vi "Complex Test.vi"() -> ()   [LabVIEW 2020, in "infolib.lvlib"]
doc: "Make a complex test of the library using premade tests/test.info."
uses:
  infolib.lvlib
  GetString.vi
  String.vi
  Get 2D String.vi
  2D String.vi
  GetTime Stamp.vi
  Time Stamp.vi
  Get 2D Time Stamp.vi
  2D Time Stamp.vi
  GetEXT.vi
  EXT.vi
  GetCXT.vi
  CXT.vi
  Get 2D EXT.vi
  2D EXT.vi
  Get 2D CXT.vi
  2D CXT.vi
  <vilib>/Utility/error.llb/Error Cluster From Error Code.vi
  <vilib>/ErrorRing/Error Ring.xnode
panel:
  in  "Test definitions and correct values":T1(array[cluster])=[{"k"="Test key, no value", "v"=[[""]], "t"="string", "s"=[]}, {"k"="Test key", "v"=[["A"]], "t"="string", "s"=[]}, {"k"="Test key, similar", "v"=[["B"]], "t"="string", "s"=[]}, {"k"="Test key, no spaces", "v"=[["C"]], "t"="string", "s"=[]}, {"k"="Test key, both spaces", "v"=[["D"]], "t"="string", "s"=[]}, {"k"="Test key, space left", "v"=[["E"]], "t"="string", "s"=[]}, {"k"="Test key, space right", "v"=[["F"]], "t"="string", "s"=[]}, {"k"="Test integer, 16 digits", "v"=[["1234567890123456"]], "t"="number", "s"=[]}, {"k"="Test floating point, 16 digits after decimal dot", "v"=[["0.1234567890123456"]], "t"="number", "s"=[]}, {"k"="Test floating point, 15 digits before decimal dot", "v"=[["123456789012345.6"]], "t"="number", "s"=[]}, {"k"="Test complex number", "v"=[["2.34+5.67i"]], "t"="compl. number", "s"=[]}, {"k"="Test imaginary number", "v"=[["8.90i"]], "t"="compl. number", "s"=[]}, {"k"="Test string, simple", "v"=[["test string"]], "t"="string", "s"=[]}, {"k"="Test string, nonletter characters", "v"=[["!@#$%^&*()-=[]{};'\"\\'\\\"\\:|,./<>?"]], "t"="string", "s"=[]}, {"k"="Test string, nonletter characters in key !@#$%^&*()-=[]{};'\"\\'\\\"\\:|,./<>?", "v"=[["in key"]], "t"="string", "s"=[]}, {"k"="Test string, UTF8 characters", "v"=[["\\u0159\\u0153\\u0414\\u03bc\\u03a9\\u211c\\u2111"]], "t"="string", "s"=[]}, {"k"="Test string, UTF8 characters in key \\u0159\\u0153\\u0414\\u03bc\\u03a9\\u211c\\u2111", "v"=[["in key"]], "t"="string", "s"=[]}, {"k"="Test time, no time zone", "v"=[["1014376332.123456"]], "t"="time", "s"=[]}, {"k"="Test time, with time zone, UTC", "v"=[["1014379932.123456"]], "t"="time", "s"=[]}, {"k"="Test time, with time zone, +10 minutes", "v"=[["1014379932.123456"]], "t"="time", "s"=[]}, {"k"="Test time, with time zone, +1 hour", "v"=[["1014379932.123456"]], "t"="time", "s"=[]}, {"k"="Test time, with time zone, -1 hour", "v"=[["1014379932.123456"]], "t"="time", "s"=[]}, {"k"="Test time, with time zone, +1:10", "v"=[["1014379932.123456"]], "t"="time", "s"=[]}, {"k"="Test time, with time zone, -1:10", "v"=[["1014379932.123456"]], "t"="time", "s"=[]}, {"k"="Test matrix, empty", "v"=[[""]], "t"="matrix number", "s"=[]}, {"k"="Test matrix, single value", "v"=[["1"]], "t"="matrix number", "s"=[]}, {"k"="Test matrix, single value, nonletter characters in key !@#$%^&*()-=[]{};'\"\\'\\\"\\:|,./<>?", "v"=[["2"]], "t"="matrix number", "s"=[]}, {"k"="Test matrix, single value, UTF8 characters in key  \\u0159\\u0153\\u0414\\u03bc\\u03a9\\u211c\\u2111", "v"=[["3"]], "t"="matrix number", "s"=[]}, {"k"="Test matrix, row numbers", "v"=[["4", "5", "6"]], "t"="matrix number", "s"=[]}, {"k"="Test matrix, column numbers", "v"=[["7"], ["8"], ["9"]], "t"="matrix number", "s"=[]}, {"k"="Test matrix", "v"=[["1.1", "2.1", "3.1"], ["4e4", "-5e5", "6e-6"], ["7.7e7", "8.123456789e1", "NaN"]], "t"="matrix number", "s"=[]}, {"k"="Test matrix complex", "v"=[["1.234", "2.345i", "3.456+4.567i"]], "t"="matrix compl. number", "s"=[]}, {"k"="Test matrix, mixed numbers and text for reading as numbers", "v"=[["1", "NaN", "2", "NaN"], ["3", "NaN", "4", "NaN"]], "t"="matrix number", "s"=[]}, {"k"="Test matrix, mixed numbers and text for reading as strings", "v"=[["11", "One", "12", "Two"], ["13", "Three", "14", "Four"]], "t"="matrix string", "s"=[]}, {"k"="Test matrix, mixed numbers and text with special characters read as numbers", "v"=[["1", "NaN", "2", "NaN"], ["3", "NaN", "4", "NaN"]], "t"="matrix number", "s"=[]}, {"k"="Test matrix, mixed numbers and text with special characters read as strings", "v"=[["11", "One;One", "12", "Two\"Two"], ["13", "Three;Three", "14", "Four\n                Four"]], "t"="matrix string", "s"=[]}, {"k"="Test matrix, time values", "v"=[["1014379932.123456", "1014383532.123456"], ["1014387132.123456", "1014390732.123456"]], "t"="matrix time", "s"=[]}, {"k"="Key for section test", "v"=[["1"]], "t"="number", "s"=[""]}, {"k"="Key for section test", "v"=[["2"]], "t"="number", "s"=["Test section"]}, {"k"="Key for section test", "v"=[["3"]], "t"="number", "s"=["Test section", "Test subsection"]}, {"k"="Key for section test", "v"=[["4"]], "t"="number", "s"=["Test section", "Test subsection", "Test subsubsection"]}, {"k"="Key for section test", "v"=[["5"]], "t"="number", "s"=["Test section", "Test subsection", "Test subsubsection", "Test subsubsubsection"]}, {"k"="Key for section test", "v"=[["6"]], "t"="number", "s"=["Test section 2"]}, {"k"="Key for section test", "v"=[["7"]], "t"="number", "s"=["Test section 2", "Test section 2"]}, {"k"="Key for section test", "v"=[["8"]], "t"="number", "s"=["Test section 2", "Test section 2", "Test section 2"]}, {"k"="Key for section test", "v"=[["9"]], "t"="number", "s"=["Test section 2", "Test section 2", "Test section 2", "Test section 2"]}, {"k"="Key for section test", "v"=[["10"]], "t"="number", "s"=["Test section, nonletter characters in key !@#$%^&*()-=[]{};'\"\\'\\\"\\:|,./<>?"]}, {"k"="Key for section test", "v"=[["11"]], "t"="number", "s"=["Test section, UTF8 characters in key \\u0159\\u0153\\u0414\\u03bc\\u03a9\\u211c\\u2111"]}, {"k"="Key for section test", "v"=[["!@#$%^&*()-=[]{};'\"\\'\\\"\\:|,./<>?"]], "t"="section", "s"=["Test section, special characters inside"]}]
  in  "Do also tmp.info?":bool=TRUE
  in  "start:":i32
  in  "end:":i32=100
  out "tmp.info: all correct?":bool
  out "tmp.info: all keys found?":bool
  out "Results of testing":T2(array[cluster])
  out "test.info: all keys found?":bool
  out "test.info: all correct?":bool
  # "k: key, v: value of correct value, t: test type, s: section(s)"
  # "For details see \"tests/info_test.m\" and \"tests/test.info\"."
  # "Do not change values in the array without changing test.info and other testing scripts (infolib_test.m)!"
  # "First run from test.info"
  # "test index, test key, key found?, test correct?"
  # "Second run from generated tmp.info"
  # "For debugging: do tests only from index"
  # "to index"
  # "(inclusive), do tmp.info"
  # "<- To make full test, set values to 0 and 100 and check tmp.info."
  # "List of bad tests, with very small impact:\n15, 16, 27, 47, 48: LV cannot handle UTF8 characters\n43: fails if tests 47 and 48 are present in tmp.info, otherwise is ok.\n30: rounding error on 17th significant place\n34,:LV cannot handle proper csv: cell \"X;X\" is considered as two cells because LV do not know apostroph enclosing\n36: rounding error on 7th decimal place of time stamp"
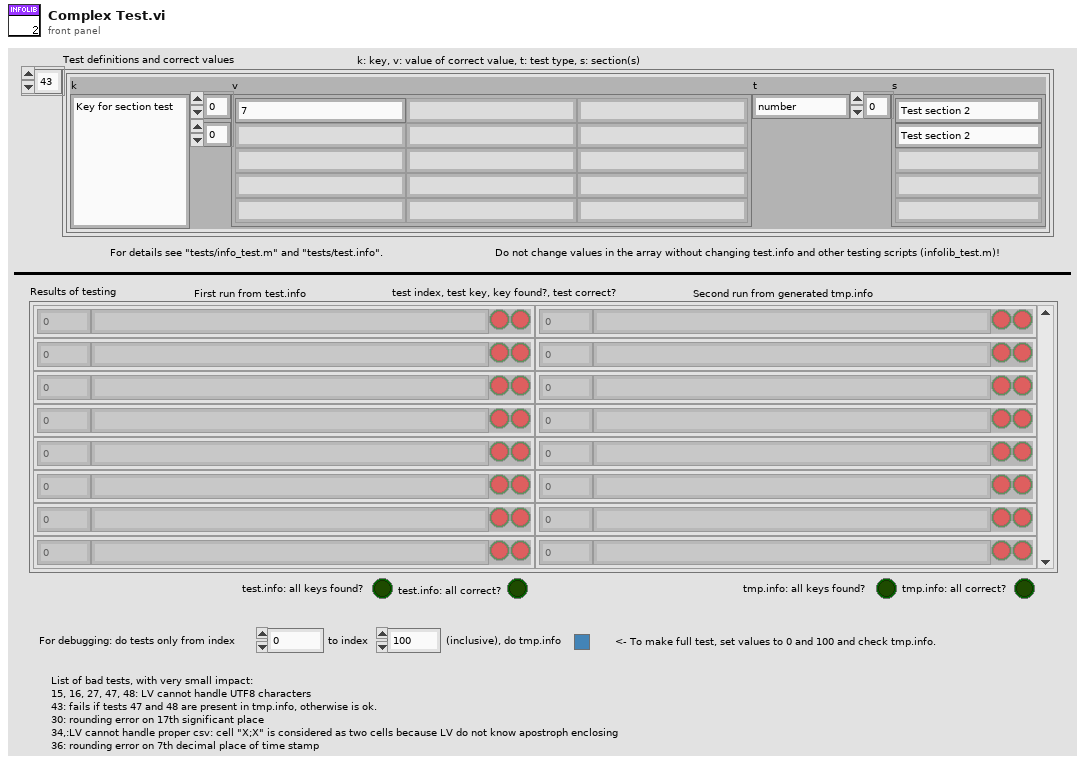
[diagram p1: front panel]
types:
  T1 = cluster{"k":string, "v":string[][], "t":string, "s":string[]}[]
  T2 = cluster{"index":i32, "key":string, "key found?":bool, "correct?":bool}[][]
  T3 = cluster{"index":i32, "key":string, "key found?":bool, "correct?":bool}
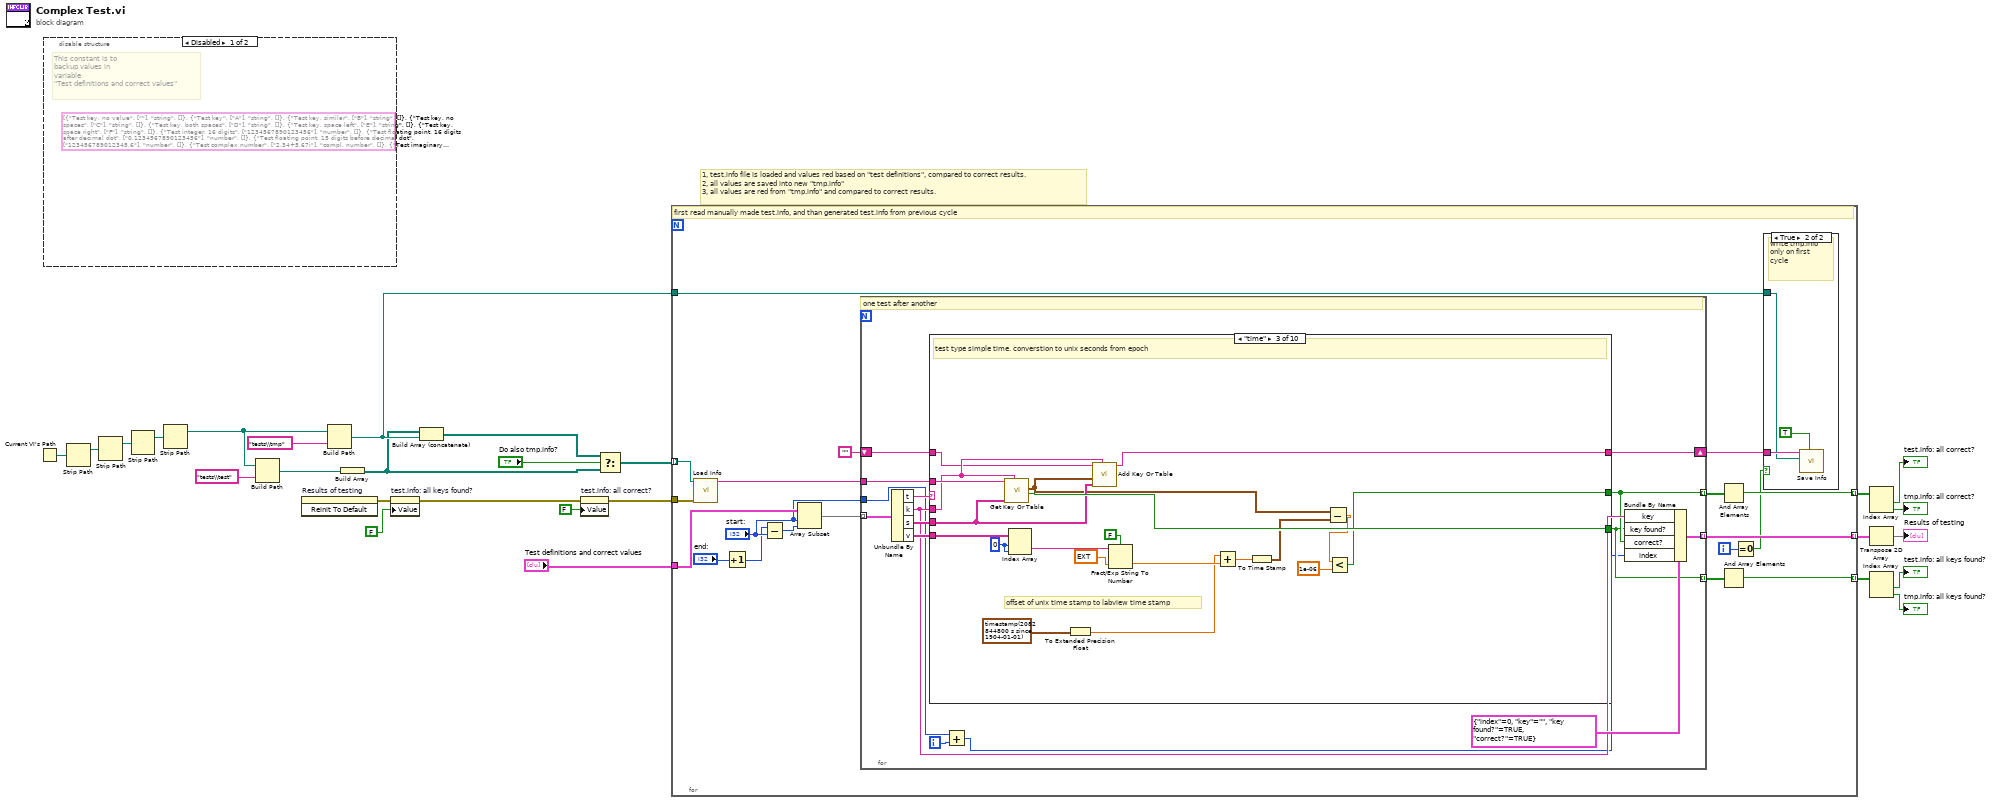
[diagram p0: block diagram]
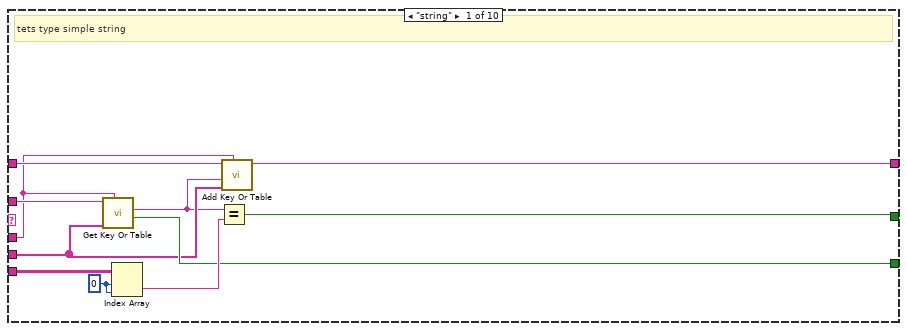
[diagram p3: hidden frame]
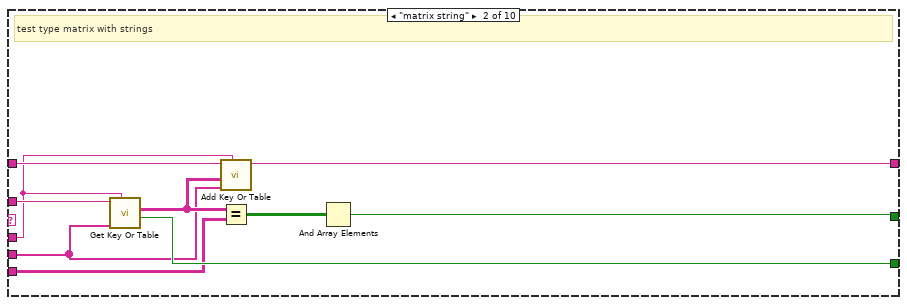
[diagram p4: hidden frame]
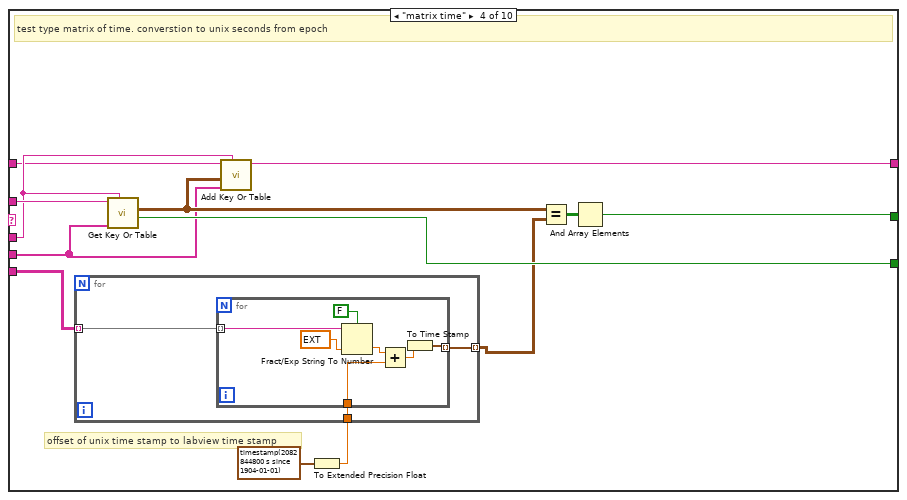
[diagram p5: hidden frame]
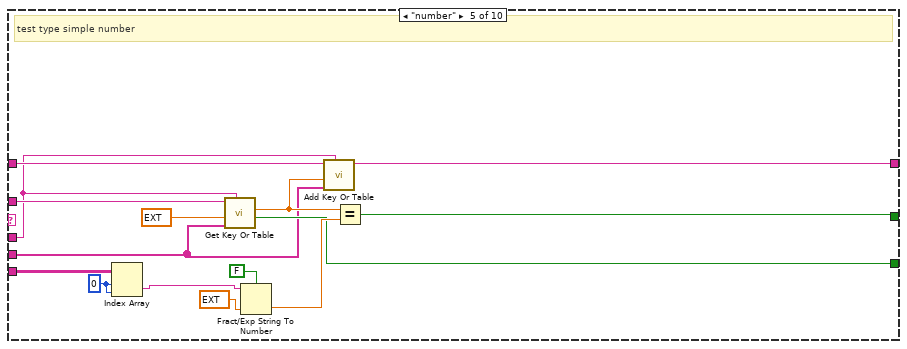
[diagram p6: hidden frame]
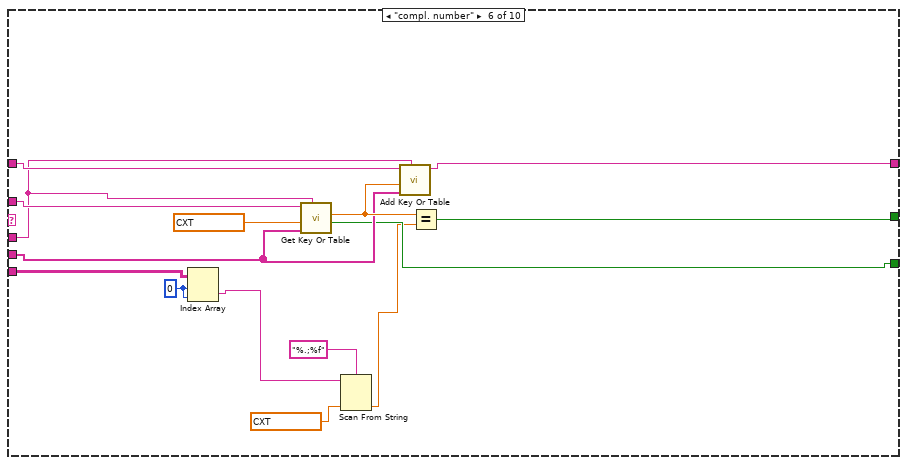
[diagram p7: hidden frame]
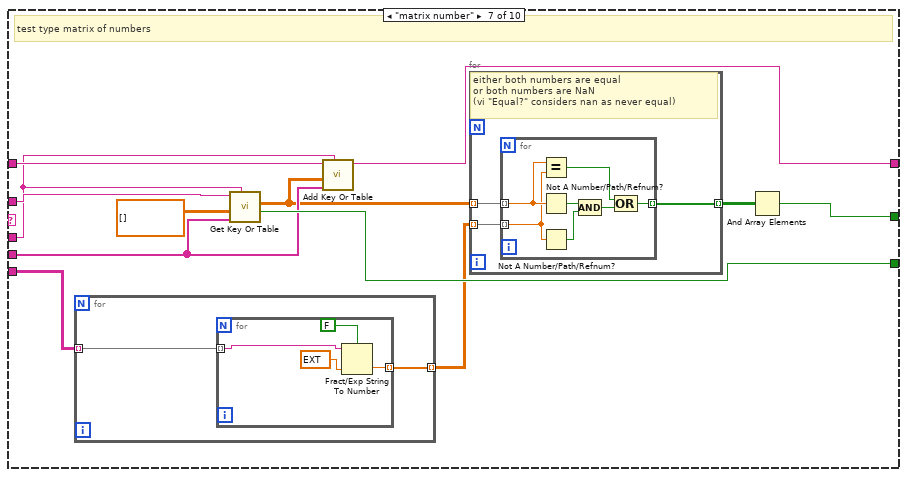
[diagram p8: hidden frame]
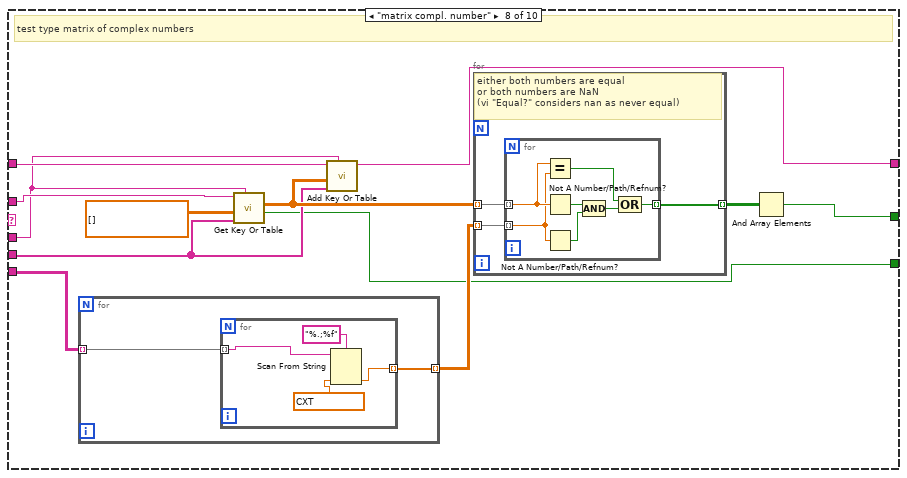
[diagram p9: hidden frame]
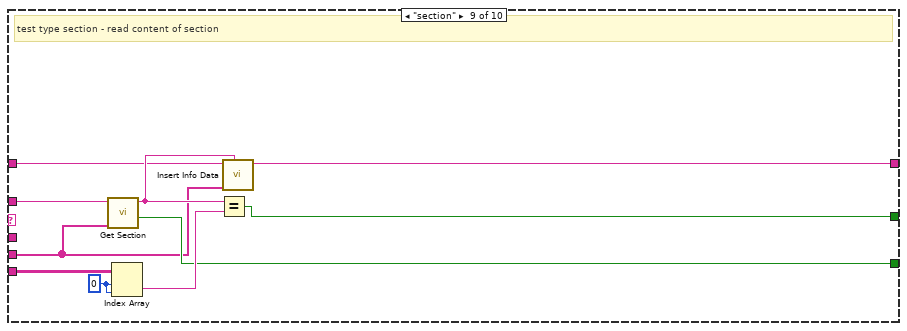
[diagram p10: hidden frame]
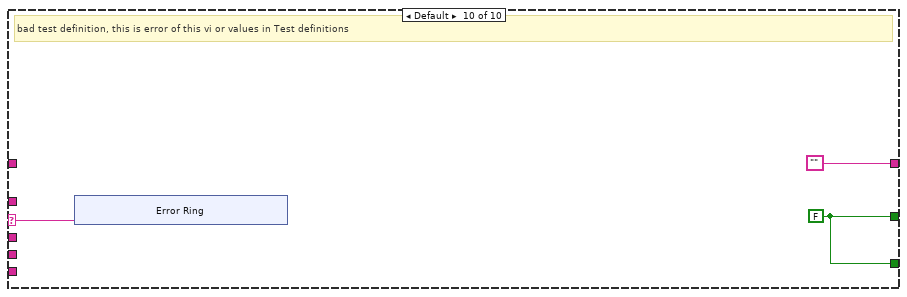
[diagram p11: hidden frame]
diagram:
  # "1, test.info file is loaded and values red based on \"test definitions\", compared to correct results.\n2, all values are saved into new \"tmp.info\"\n3, all values are red from \"tmp.info\" and compared to correct results."
  n1 = Current VI's Path() -> (path=w15:path)
  n2 = disable-structure shown="Disabled" {
    frame Disabled {
      (unwired) T1 [{"k"="Test key, no value", "v"=[[""]], "t"="string", "s"=[]}, {"k"="Test key", "v"=[["A"]], "t"="string", "s"=[]}, {"k"="Test key, similar", "v"=[["B"]], "t"="string", "s"=[]}, {"k"="Test key, no spaces", "v"=[["C"]], "t"="string", "s"=[]}, {"k"="Test key, both spaces", "v"=[["D"]], "t"="string", "s"=[]}, {"k"="Test key, space left", "v"=[["E"]], "t"="string", "s"=[]}, {"k"="Test key, space right", "v"=[["F"]], "t"="string", "s"=[]}, {"k"="Test integer, 16 digits", "v"=[["1234567890123456"]], "t"="number", "s"=[]}, {"k"="Test floating point, 16 digits after decimal dot", "v"=[["0.1234567890123456"]], "t"="number", "s"=[]}, {"k"="Test floating point, 15 digits before decimal dot", "v"=[["123456789012345.6"]], "t"="number", "s"=[]}, {"k"="Test complex number", "v"=[["2.34+5.67i"]], "t"="compl. number", "s"=[]}, {"k"="Test imaginary number", "v"=[["8.90i"]], "t"="compl. number", "s"=[]}, {"k"="Test string, simple", "v"=[["test string"]], "t"="string", "s"=[]}, {"k"="Test string, nonletter characters", "v"=[["!@#$%^&*()-=[]{};'\"\\'\\\"\\:|,./<>?"]], "t"="string", "s"=[]}, {"k"="Test string, nonletter characters in key !@#$%^&*()-=[]{};'\"\\'\\\"\\:|,./<>?", "v"=[["in key"]], "t"="string", "s"=[]}, {"k"="Test string, UTF8 characters", "v"=[["\\u0159\\u0153\\u0414\\u03bc\\u03a9\\u211c\\u2111"]], "t"="string", "s"=[]}, {"k"="Test string, UTF8 characters in key \\u0159\\u0153\\u0414\\u03bc\\u03a9\\u211c\\u2111", "v"=[["in key"]], "t"="string", "s"=[]}, {"k"="Test time, no time zone", "v"=[["1014376332.123456"]], "t"="time", "s"=[]}, {"k"="Test time, with time zone, UTC", "v"=[["1014379932.123456"]], "t"="time", "s"=[]}, {"k"="Test time, with time zone, +10 minutes", "v"=[["1014379932.123456"]], "t"="time", "s"=[]}, {"k"="Test time, with time zone, +1 hour", "v"=[["1014379932.123456"]], "t"="time", "s"=[]}, {"k"="Test time, with time zone, -1 hour", "v"=[["1014379932.123456"]], "t"="time", "s"=[]}, {"k"="Test time, with time zone, +1:10", "v"=[["1014379932.123456"]], "t"="time", "s"=[]}, {"k"="Test time, with time zone, -1:10", "v"=[["1014379932.123456"]], "t"="time", "s"=[]}, {"k"="Test matrix, empty", "v"=[[""]], "t"="matrix number", "s"=[]}, {"k"="Test matrix, single value", "v"=[["1"]], "t"="matrix number", "s"=[]}, {"k"="Test matrix, single value, nonletter characters in key !@#$%^&*()-=[]{};'\"\\'\\\"\\:|,./<>?", "v"=[["2"]], "t"="matrix number", "s"=[]}, {"k"="Test matrix, single value, UTF8 characters in key  \\u0159\\u0153\\u0414\\u03bc\\u03a9\\u211c\\u2111", "v"=[["3"]], "t"="matrix number", "s"=[]}, {"k"="Test matrix, row numbers", "v"=[["4", "5", "6"]], "t"="matrix number", "s"=[]}, {"k"="Test matrix, column numbers", "v"=[["7"], ["8"], ["9"]], "t"="matrix number", "s"=[]}, {"k"="Test matrix", "v"=[["1.1", "2.1", "3.1"], ["4e4", "-5e5", "6e-6"], ["7.7e7", "8.123456789e1", "NaN"]], "t"="matrix number", "s"=[]}, {"k"="Test matrix complex", "v"=[["1.234", "2.345i", "3.456+4.567i"]], "t"="matrix compl. number", "s"=[]}, {"k"="Test matrix, mixed numbers and text for reading as numbers", "v"=[["1", "NaN", "2", "NaN"], ["3", "NaN", "4", "NaN"]], "t"="matrix number", "s"=[]}, {"k"="Test matrix, mixed numbers and text for reading as strings", "v"=[["11", "One", "12", "Two"], ["13", "Three", "14", "Four"]], "t"="matrix string", "s"=[]}, {"k"="Test matrix, mixed numbers and text with special characters read as numbers", "v"=[["1", "NaN", "2", "NaN"], ["3", "NaN", "4", "NaN"]], "t"="matrix number", "s"=[]}, {"k"="Test matrix, mixed numbers and text with special characters read as strings", "v"=[["11", "One;One", "12", "Two\"Two"], ["13", "Three;Three", "14", "Four\n                Four"]], "t"="matrix string", "s"=[]}, {"k"="Test matrix, time values", "v"=[["1014379932.123456", "1014379932.123456+1*3600"], ["1014379932.123456+2*3600", "1014379932.123456+3*3600"]], "t"="matrix time", "s"=[]}, {"k"="Key for section test", "v"=[["1"]], "t"="number", "s"=[""]}, {"k"="Key for section test", "v"=[["2"]], "t"="number", "s"=["Test section"]}, {"k"="Key for section test", "v"=[["3"]], "t"="number", "s"=["Test section", "Test subsection"]}, {"k"="Key for section test", "v"=[["4"]], "t"="number", "s"=["Test section", "Test subsection", "Test subsubsection"]}, {"k"="Key for section test", "v"=[["5"]], "t"="number", "s"=["Test section", "Test subsection", "Test subsubsection", "Test subsubsubsection"]}, {"k"="Key for section test", "v"=[["6"]], "t"="number", "s"=["Test section 2"]}, {"k"="Key for section test", "v"=[["7"]], "t"="number", "s"=["Test section 2", "Test section 2"]}, {"k"="Key for section test", "v"=[["8"]], "t"="number", "s"=["Test section 2", "Test section 2", "Test section 2"]}, {"k"="Key for section test", "v"=[["9"]], "t"="number", "s"=["Test section 2", "Test section 2", "Test section 2", "Test section 2"]}, {"k"="Key for section test", "v"=[["10"]], "t"="number", "s"=["Test section, nonletter characters in key !@#$%^&*()-=[]{};'\"\\'\\\"\\:|,./<>?"]}, {"k"="Key for section test", "v"=[["11"]], "t"="number", "s"=["Test section, UTF8 characters in key \\u0159\\u0153\\u0414\\u03bc\\u03a9\\u211c\\u2111"]}, {"k"="Key for section test", "v"=[["!@#$%^&*()-=[]{};'\"\\'\\\"\\:|,./<>?"]], "t"="section", "s"=["Test section, special characters inside"]}] ("Test definitions and correct values")
      # "This constant is to\nbackup values in\nvariable\n\"Test definitions and correct values\""
    }
    frame Enabled {
    }
  }
  n3 = Strip Path(path=w15) -> (stripped path=w14:path)  [unwired: 1 out]
  n4 = Strip Path(path=w14) -> (stripped path=w13:path)  [unwired: 1 out]
  n5 = Strip Path(path=w13) -> (stripped path=w12:path)  [unwired: 1 out]
  n6 = Strip Path(path=w12) -> (stripped path=w11:path)  [unwired: 1 out]
  n7 = Build Path(base path=w11, name or relative path="tests\\test") -> (appended path=w3:path)
  n8 = invoke on="Results of testing" class="Arr (strict)" method="Reinit To Default"() -> (error out=w8:errorcluster)  [unwired: 3 in, 2 out]
  n9 = Build Path(base path=w11, name or relative path="tests\\tmp") -> (appended path=w7:path)
  n10 = Build Array(w3) -> (w2:path[])
  n11 = property on="test.info: all keys found?" class="Bool (strict)"(error in=w8, "Value"=FALSE ("All keys found?")) -> (error out=w27:errorcluster)  [unwired: 1 in, 1 out]
  n12 = Build Array (concatenate)(w2, w7) -> (w4:path[])
  n13 = property on="test.info: all correct?" class="Bool (strict)"(error in=w27, "Value"=FALSE ("All correct?")) -> (error out=w26:errorcluster)  [unwired: 1 in, 1 out]
  n14 = Select(t=w4, s="Do also tmp.info?", f=w2) -> (s? t:f=w6:path[])
  n15 = for {
    tunnel: "Test definitions and correct values" -> [w33]
    tunnel: w6 -> [w46] mode=indexing
    tunnel: w26 -> [w44]
    tunnel: [w43] -> w10 mode=indexing
    tunnel: [w41] -> w17 mode=indexing
    tunnel: [w39] -> w21 mode=indexing
    tunnel: w7 -> [w34]
    i -> [w37]
    # "first read manually made test.info, and than generated test.info from previous cycle"
    n16 = call "Load Info.vi"("error in"=w44, "filename"=w46) -> ("info data"=w45:string)  [unwired: 8 in, 1 out]
    n17 = Increment(x="end:") -> (x+1=w28:i32)
    n18 = Subtract(x=w28, y="start:") -> (x-y=w30:i32)
    n19 = Array Subset(array=w33, index="start:", length=w30) -> (w32:T1)
    n20 = for {
      tunnel: w32 -> [w64] mode=indexing
      tunnel: w45 -> [w63]
      tunnel: [w57] -> w43 mode=indexing
      tunnel: [w56] -> w42 mode=indexing
      tunnel: [w55] -> w40 mode=indexing
      shift-right: [w53] -> w35
      shift-left: "" -> [w54]
      tunnel: "start:" -> [w51]
      i -> [w52]
      # "one test after another"
      n21 = Unbundle By Name(w64) -> ("t"=w62:string, "k"=w58:string, "s"=w61:string[], "v"=w60:string[][])
      n22 = case shown="\"time\"" w62 {
        selector: w62 -> [_ _ _ _ _ _ _ _ _ w226]
        tunnel: w58 -> [w67 w79 w96 w111 w134 w154 w163 w192 _ _]
        tunnel: w63 -> [w75 w85 w105 w118 w143 w155 w170 w193 w224 _]
        tunnel: w61 -> [w69 w77 w95 w108 w132 w152 w162 w191 w216 _]
        tunnel: w60 -> [w74 w83 w104 w115 w142 w153 w167 w190 w223 _]
        tunnel: [w72 w81 w86 w113 w141 w151 w166 w187 w220 w227] -> w56
        tunnel: [w71 w84 w103 w117 w137 w149 w169 w189 w219 w227] -> w55
        tunnel: w54 -> [w70 w80 w94 w110 w135 w156 w165 w194 w217 _]
        tunnel: [w66 w76 w93 w109 w131 w150 w164 w188 w215 ""] -> w53
        frame "string" {
          w65 = 0 ("index (row)")
          # "tets type simple string"
          n23 = call-poly "Get Key Or Table.vi"("key description"=w67, "sections"=w69, "info data"=w75) -> ("key found?"=w71:bool, "value"=w68:string)  [unwired: 5 in, 2 out]
          n24 = Index Array(array=w74, index (row)=w65, index (col)=w65) -> (element=w73:string)
          n25 = Equal?(x=w68, y=w73) -> (x = y?=w72:bool)
          n26 = call-poly "Add Key Or Table.vi"("key description"=w67, "sections"=w69, "string"=w68, "info data"=w70) -> ("info data out"=w66:string)  [unwired: 6 in, 1 out]
        }
        frame "matrix string" {
          # "test type matrix with strings"
          n27 = call-poly "Get Key Or Table.vi"("key description"=w79, "sections"=w77, "info data"=w85) -> ("key found?"=w84:bool, "value"=w78:string[][])  [unwired: 5 in, 2 out]
          n28 = call-poly "Add Key Or Table.vi"("key description"=w79, "sections"=w77, "string"=w78, "info data"=w80) -> ("info data out"=w76:string)  [unwired: 6 in, 1 out]
          n29 = Equal?(x=w78, y=w83) -> (x = y?=w82:bool[][])
          n30 = And Array Elements(Boolean array=w82) -> (logical AND=w81:bool)
        }
        frame "time" {
          w92 = 0 ("index (row)")
          # "offset of unix time stamp to labview time stamp"
          # "test type simple time. converstion to unix seconds from epoch"
          n31 = call-poly "Get Key Or Table.vi"("key description"=w96, "sections"=w95, "info data"=w105) -> ("key found?"=w103:bool, "value"=w89:timestamp)  [unwired: 5 in, 2 out]
          n32 = Index Array(array=w104, index (row)=w92, index (col)=w92) -> (element=w101:string)
          n33 = To Extended Precision Float(1:timestamp(2082844800 s since 1904-01-01)) -> (0:w99:ext)
          n34 = call-poly "Add Key Or Table.vi"("key description"=w96, "sections"=w95, "time stamp"=w89, "info data"=w94) -> ("info data out"=w93:string)  [unwired: 6 in, 1 out]
          n35 = Fract/Exp String To Number(use system decimal point (T)=FALSE, string=w101, default (0 dbl)=ext nan ("default (0 DBL)")) -> (number=w100:ext)  [unwired: 1 in, 1 out]
          n36 = Add(x=w99, y=w100) -> (x+y=w97:ext)
          n37 = To Time Stamp(1:w97) -> (0:w90:timestamp)
          n38 = Subtract(x=w89, y=w90) -> (x-y=w88:dbl)
          n39 = Less?(x=w88, y=1e-06) -> (x < y?=w86:bool)
        }
        frame "matrix time" {
          # "offset of unix time stamp to labview time stamp"
          # "test type matrix of time. converstion to unix seconds from epoch"
          n40 = call-poly "Get Key Or Table.vi"("key description"=w111, "sections"=w108, "info data"=w118) -> ("key found?"=w117:bool, "value"=w112:timestamp[][])  [unwired: 5 in, 2 out]
          n41 = call-poly "Add Key Or Table.vi"("key description"=w111, "sections"=w108, "time stamp"=w112, "info data"=w110) -> ("info data out"=w109:string)  [unwired: 6 in, 1 out]
          n42 = To Extended Precision Float(1:timestamp(2082844800 s since 1904-01-01)) -> (0:w106:ext)
          n43 = for {
            tunnel: [w121] -> w107 mode=indexing
            tunnel: w115 -> [w120] mode=indexing
            tunnel: w106 -> [w119]
            n44 = for {
              tunnel: [w123] -> w121 mode=indexing
              tunnel: w120 -> [w127] mode=indexing
              tunnel: w119 -> [w122]
              n45 = Fract/Exp String To Number(use system decimal point (T)=FALSE, string=w127, default (0 dbl)=ext nan ("default (0 DBL)")) -> (number=w125:ext)  [unwired: 1 in, 1 out]
              n46 = Add(x=w125, y=w122) -> (x+y=w124:ext)
              n47 = To Time Stamp(1:w124) -> (0:w123:timestamp)
            }
          }
          n48 = Equal?(x=w112, y=w107) -> (x = y?=w114:bool[][])
          n49 = And Array Elements(Boolean array=w114) -> (logical AND=w113:bool)
        }
        frame "number" {
          w130 = 0 ("index (row)")
          # "test type simple number"
          n50 = Index Array(array=w142, index (row)=w130, index (col)=w130) -> (element=w140:string)
          n51 = call-poly "Get Key Or Table.vi"("key description"=w134, "sections"=w132, "numeric"=ext nan, "info data"=w143) -> ("key found?"=w137:bool, "value"=w133:ext)  [unwired: 4 in, 2 out]
          n52 = Fract/Exp String To Number(use system decimal point (T)=FALSE, string=w140, default (0 dbl)=ext nan ("default (0 DBL)")) -> (number=w139:ext)  [unwired: 1 in, 1 out]
          n53 = call-poly "Add Key Or Table.vi"("key description"=w134, "sections"=w132, "numeric"=w133, "info data"=w135) -> ("info data out"=w131:string)  [unwired: 6 in, 1 out]
          n54 = Equal?(x=w133, y=w139) -> (x = y?=w141:bool)
        }
        frame "compl. number" {
          w157 = 0 ("index (row)")
          n55 = Index Array(array=w153, index (row)=w157, index (col)=w157) -> (element=w146:string)
          n56 = call-poly "Get Key Or Table.vi"("key description"=w154, "sections"=w152, "numeric"=cxt nan+nani, "info data"=w155) -> ("key found?"=w149:bool, "value"=w158:cxt)  [unwired: 4 in, 2 out]
          n57 = Scan From String(format string="%.;%f", input string=w146, default 1=cxt nan+nani ("numeric")) -> (output 1=w145:cxt)  [unwired: 2 in, 3 out]
          n58 = call-poly "Add Key Or Table.vi"("key description"=w154, "sections"=w152, "numeric"=w158, "info data"=w156) -> ("info data out"=w150:string)  [unwired: 6 in, 1 out]
          n59 = Equal?(x=w158, y=w145) -> (x = y?=w151:bool)
        }
        frame "matrix number" {
          # "test type matrix of numbers"
          n60 = for {
            tunnel: w167 -> [w182] mode=indexing
            tunnel: [w181] -> w160 mode=indexing
            n61 = for {
              tunnel: w182 -> [w185] mode=indexing
              tunnel: [w184] -> w181 mode=indexing
              n62 = Fract/Exp String To Number(use system decimal point (T)=FALSE, string=w185, default (0 dbl)=ext nan ("default (0 DBL)")) -> (number=w184:ext)  [unwired: 1 in, 1 out]
            }
          }
          n63 = call-poly "Get Key Or Table.vi"("key description"=w163, "sections"=w162, "numeric"=ext[][] [], "info data"=w170) -> ("key found?"=w169:bool, "value"=w161:ext[][])  [unwired: 4 in, 2 out]
          n64 = call-poly "Add Key Or Table.vi"("key description"=w163, "sections"=w162, "numeric"=w161, "info data"=w165) -> ("info data out"=w164:string)  [unwired: 6 in, 1 out]
          n65 = for {
            tunnel: w161 -> [w173] mode=indexing
            tunnel: w160 -> [w172] mode=indexing
            tunnel: [w171] -> w159 mode=indexing
            # "either both numbers are equal\nor both numbers are NaN\n(vi \"Equal?\" considers nan as never equal)"
            n66 = for {
              tunnel: w173 -> [w180] mode=indexing
              tunnel: w172 -> [w179] mode=indexing
              tunnel: [w174] -> w171 mode=indexing
              n67 = Equal?(x=w180, y=w179) -> (x = y?=w175:bool)
              n68 = Not A Number/Path/Refnum?(number/path/refnum=w180) -> (NaN/Path/Refnum?=w176:bool)
              n69 = Not A Number/Path/Refnum?(number/path/refnum=w179) -> (NaN/Path/Refnum?=w177:bool)
              n70 = Compound Arithmetic op=AND(w176, w177) -> (w178:bool)
              n71 = Compound Arithmetic op=OR(w175, w178) -> (w174:bool)
            }
          }
          n72 = And Array Elements(Boolean array=w159) -> (logical AND=w166:bool)
        }
        frame "matrix compl. number" {
          # "test type matrix of complex numbers"
          n73 = for {
            tunnel: w190 -> [w210] mode=indexing
            tunnel: [w209] -> w197 mode=indexing
            n74 = for {
              tunnel: w210 -> [w211] mode=indexing
              tunnel: [w212] -> w209 mode=indexing
              n75 = Scan From String(format string="%.;%f", input string=w211, default 1=cxt nan+nani ("numeric")) -> (output 1=w212:cxt)  [unwired: 2 in, 3 out]
            }
          }
          n76 = call-poly "Get Key Or Table.vi"("key description"=w192, "sections"=w191, "numeric"=cxt[][] [], "info data"=w193) -> ("key found?"=w189:bool, "value"=w198:cxt[][])  [unwired: 4 in, 2 out]
          n77 = call-poly "Add Key Or Table.vi"("key description"=w192, "sections"=w191, "numeric"=w198, "info data"=w194) -> ("info data out"=w188:string)  [unwired: 6 in, 1 out]
          n78 = for {
            tunnel: w198 -> [w201] mode=indexing
            tunnel: w197 -> [w200] mode=indexing
            tunnel: [w199] -> w196 mode=indexing
            # "either both numbers are equal\nor both numbers are NaN\n(vi \"Equal?\" considers nan as never equal)"
            n79 = for {
              tunnel: w201 -> [w208] mode=indexing
              tunnel: w200 -> [w207] mode=indexing
              tunnel: [w202] -> w199 mode=indexing
              n80 = Equal?(x=w208, y=w207) -> (x = y?=w203:bool)
              n81 = Not A Number/Path/Refnum?(number/path/refnum=w208) -> (NaN/Path/Refnum?=w204:bool)
              n82 = Not A Number/Path/Refnum?(number/path/refnum=w207) -> (NaN/Path/Refnum?=w205:bool)
              n83 = Compound Arithmetic op=AND(w204, w205) -> (w206:bool)
              n84 = Compound Arithmetic op=OR(w203, w206) -> (w202:bool)
            }
          }
          n85 = And Array Elements(Boolean array=w196) -> (logical AND=w187:bool)
        }
        frame "section" {
          w222 = 0 ("index (row)")
          # "test type section - read content of section"
          n86 = call "Get Section.vi"("sections"=w216, "info data"=w224) -> ("exist"=w219:bool, "section part"=w218:string)  [unwired: 7 in, 1 out]
          n87 = Index Array(array=w223, index (row)=w222, index (col)=w222) -> (element=w221:string)
          n88 = Equal?(x=w218, y=w221) -> (x = y?=w220:bool)
          n89 = call "Insert Info Data.vi"("info data to insert"=w218, "sections"=w216, "info data"=w217) -> ("info data out"=w215:string)  [unwired: 7 in, 1 out]
        }
        frame Default {
          w227 = FALSE
          # "bad test definition, this is error of this vi or values in Test definitions"
          n90 = xnode "Error Ring"("parameter 0"=w226) -> ()  [unwired: 1 out]
        }
      }
      n91 = Add(x=w51, y=w52) -> (x+y=w50:i32)
      n92 = Bundle By Name(cluster=T3 {"index"=0, "key"="", "key found?"=TRUE, "correct?"=TRUE}, "key"=w58, "key found?"=w55, "correct?"=w56, "index"=w50) -> (w57:T3)
    }
    n93 = And Array Elements(Boolean array=w42) -> (logical AND=w41:bool)
    n94 = And Array Elements(Boolean array=w40) -> (logical AND=w39:bool)
    n95 = Equal To 0?(x=w37) -> (x = 0?=w36:bool)
    n96 = case shown="True" w36 {
      tunnel: w35 -> [_ w49]
      tunnel: w34 -> [_ w47]
      frame False {
      }
      frame True {
        # "write tmp.info\nonly on first\ncycle"
        n97 = call "Save Info.vi"("Overwrite? (T)"=TRUE, "filename"=w47, "info data"=w49) -> ()  [unwired: 8 in, 1 out]
      }
    }
  }
  n98 = Index Array(array=w17) -> (element #1=→"test.info: all correct?":bool, element #2=→"tmp.info: all correct?":bool)  [unwired: 2 in]
  n99 = Transpose 2D Array(2D array=w10) -> (transposed array=→"Results of testing":T2)
  n100 = Index Array(array=w21) -> (element #1=→"test.info: all keys found?":bool, element #2=→"tmp.info: all keys found?":bool)  [unwired: 2 in]
